vi "FTW-CodeGen-Prototype.vi"(0 "REPLACE_Actor Instance Configuration":string="{\n  \"Identity\": \"ActorName\",\n  \"InboxAddress\": \"tcp://127.0.0.1:*\",\n  \"SupervisorAddress\": \"\",\n  \"DebugEnableInboxLogging\": false,\n  \"DebugEnableJobLogging\": false,\n  \"DebugShowPanel\": false\n}", 2 "ADAPT_Actor Instance Interface":refnum<vi>, 5 "REPLACE_Launch Actor from Filepath":path=path "", 11 "REPLACE_error in":errorcluster) -> (4 "REPLACE_FTW Actor Connector":T1, 6 "REPLACE_Instance Inbox Address":string, 8 "REPLACE_Instance VI Clone Name":string, 15 "REPLACE_error out":errorcluster)   [LabVIEW 2015, in "FTW-Actor-Spawn.xnode"]
uses:
  FTW-Actor-Spawn.xnode
  src/core/type/FTW-Type-Actor-Connector.ctl
  src/error/FTW-ERR-ThrowError.vi
  src/reflection/FTW-Reflection-Type.vi
  src/error/FTW-ERR-NoErrorConstant.vi
  src/error/FTW-ERR-StatusException.vi
  src/error/FTW-ERR-CallChain.vi
  src/string/FTW-STR-ReplaceWhitespace.vi
  src/reflection/FTW-Reflection-Array.vi
  src/string/FTW-STR-Array-Delimit.vi
  src/error/FTW-ERR-Clear.vi
  src/regex/FTW-Regex-ReplaceAll.vi
  lib/FTW-KernelFilepath.vi
  src/json/core/FTW-JSON-Core-EncodingFlags.vi
  json/fetch/FTW-JSON-Core-GetFlattenedValue.vi
  FTW-JSON-Fetch.xnode
panel:
  # "Inputs"
  # "Outputs"
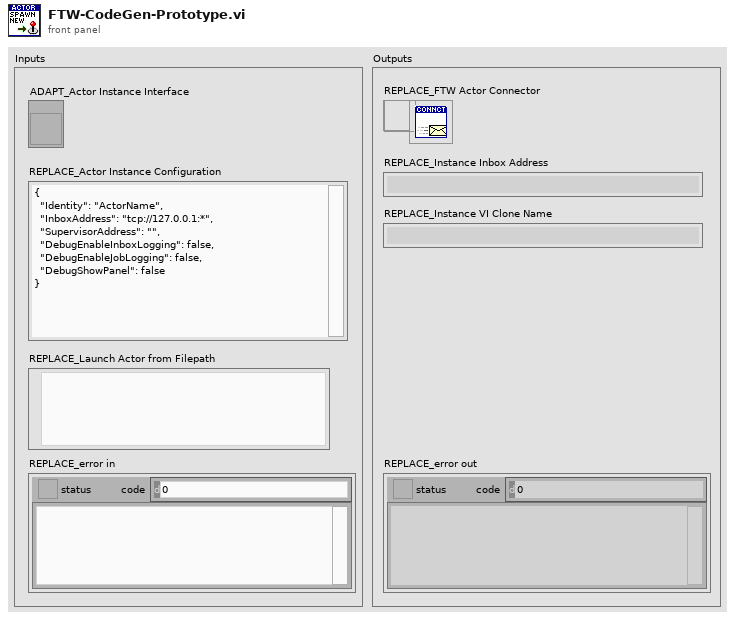
[diagram p1: front panel]
types:
  T1 = typedef "FTW-Type-Actor-Connector.ctl" = refnum<data-value>
  T2 = cluster{"FTW-PrimaryInboxAddress":string, "FTW-InstanceCloneName":string}
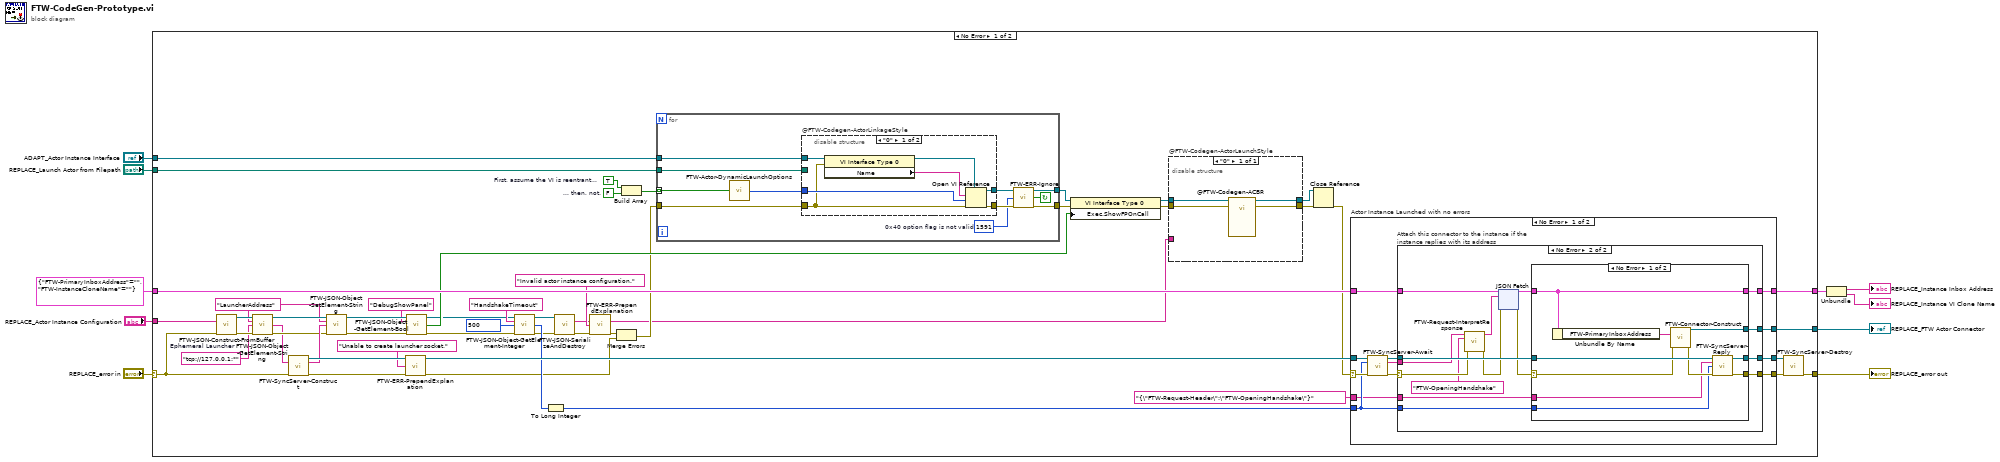
[diagram p0: block diagram]
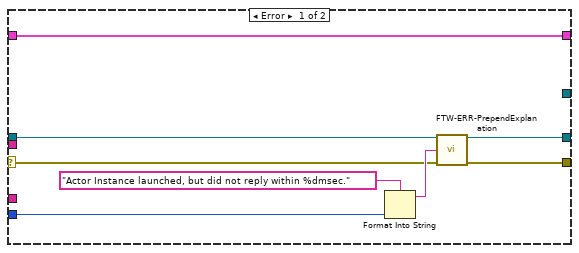
[diagram p2: hidden frame]
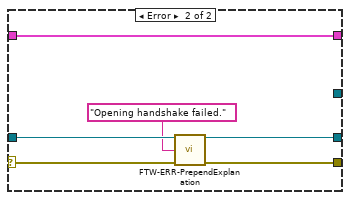
[diagram p3: hidden frame]
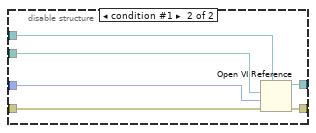
[diagram p5: hidden frame]
diagram:
  n1 = case shown="No Error" "REPLACE_error in" {
    selector: "REPLACE_error in" -> [w37 w202]
    tunnel: [w57 w202] -> w8
    tunnel: [w60 _] -> w9
    tunnel: "REPLACE_Actor Instance Configuration" -> [w40 _]
    tunnel: T2 {"FTW-PrimaryInboxAddress"="", "FTW-InstanceCloneName"=""} -> [w55 w201]
    tunnel: [w54 w201] -> w6
    tunnel: "ADAPT_Actor Instance Interface" -> [w44 _]
    tunnel: "REPLACE_Launch Actor from Filepath" -> [w41 _]
    frame No Error {
      w49 = FALSE  # ... then, not.
      w48 = TRUE  # First, assume the VI is reentrant...
      w13 = "tcp://127.0.0.1:*"  # Ephemeral Launcher
      w11 = "LauncherAddress" ("Key")
      n2 = call "FTW-JSON-Construct-FromBuffer.vi"("JSON String (UTF-8)"=w40, "error in"=w37) -> ("JSON Object"=w17:refnum<data-value>, "error out"=w15:errorcluster)  [unwired: 12 in]
      n3 = call "FTW-JSON-Object-GetElement-String.vi"("JSON Object"=w17, "Key"=w11, "Default Value"=w13, "error in"=w15) -> ("JSON Object out"=w16:refnum<data-value>, "Value"=w12:string, "error out"=w14:errorcluster)  [unwired: 8 in, 1 out]
      n4 = call "FTW-SyncServer-Construct.vi"("Instance Inbox Address"=w12, "error in"=w37) -> ("FTW Synchronous Server"=w56:refnum<data-value>, "Resolved Inbox Address"=w39:string, "error out"=w24:errorcluster)  [unwired: 11 in]
      n5 = call "FTW-JSON-Object-SetElement-String.vi"("JSON Object"=w16, "Key"=w11, "Value"=w39, "error in"=w14) -> ("JSON Object out"=w38:refnum<data-value>, "error out"=w36:errorcluster)  [unwired: 10 in]
      n6 = call "FTW-ERR-PrependExplanation.vi"("Exception Information"="Unable to create launcher socket.", "error in"=w24) -> ("error out"=w23:errorcluster)  [unwired: 13 in]
      n7 = call "FTW-JSON-Object-GetElement-Bool.vi"("JSON Object"=w38, "Key"="DebugShowPanel", "error in"=w36) -> ("JSON Object out"=w32:refnum<data-value>, "Value"=w34:bool, "error out"=w31:errorcluster)  [unwired: 9 in, 1 out]
      n8 = call "FTW-JSON-Object-GetElement-Integer.vi"("JSON Object"=w32, "Key"="HandshakeTimeout", "Default Value"=i64 500, "error in"=w31) -> ("JSON Object out"=w27:refnum<data-value>, "Value"=w30:i64, "error out"=w26:errorcluster)  [unwired: 8 in, 1 out]
      n9 = To Long Integer(number=w30) -> (32bit integer=w29:i32)
      n10 = call "FTW-JSON-SerializeAndDestroy.vi"("JSON Object"=w27, "error in"=w26) -> ("JSON String (UTF-8)"=w18:string, "error out"=w21:errorcluster)  [unwired: 12 in]
      n11 = call "FTW-ERR-PrependExplanation.vi"("Exception Information"="Invalid actor instance configuration.", "error in"=w21) -> ("error out"=w20:errorcluster)  [unwired: 13 in]
      n12 = Merge Errors(w20, w23) -> (w25:errorcluster)
      n13 = Build Array(w48, w49) -> (w50:bool[])
      n14 = for {
        tunnel: w44 -> [w187]
        tunnel: [w185] -> w46
        tunnel: [w181] -> w47
        tunnel: w50 -> [w184] mode=indexing
        tunnel: w25 -> [w183]
        tunnel: w41 -> [w182]
        stop <- w179 continue-if-true
        w178 = 1591  # 0x40 option flag is not valid
        n15 = call "FTW-Actor-DynamicLaunchOptions.vi"("Reentrant?"=w184) -> ("Open VI Ref Options"=w186:i32)
        n16 = disable-structure "@FTW-Codegen-ActorLinkageStyle" shown="\"0\"" {
          disable-tunnel: w187 -> [w194 w200]
          disable-tunnel: w186 -> [w193 w199]
          disable-tunnel: [w192 w198] -> w185
          disable-tunnel: w183 -> [w191 w197]
          disable-tunnel: [w190 w196] -> w180
          disable-tunnel: w182 -> [_ w195]
          frame condition #0 (active) {
            n17 = property class="VI Interface Type 0"(reference=w194, error in=w191) -> (reference out=w189:refnum<vi>, "Name"=w188:string)  [unwired: 1 out]
            n18 = Open VI Reference(type specifier VI Refnum (for type only)=w189, vi path=w188, options=w193, error in (no error)=w191) -> (vi reference=w192:refnum<vi>, error out=w190:errorcluster)  [unwired: 2 in]
          }
          frame condition #1 {
            n19 = Open VI Reference(type specifier VI Refnum (for type only)=w200, vi path=w195, options=w199, error in (no error)=w197) -> (vi reference=w198:refnum<vi>, error out=w196:errorcluster)  [unwired: 2 in]
          }
        }
        n20 = call "FTW-ERR-Ignore.vi"("Error Code"=w178, "error in"=w180) -> ("Error Cleared?"=w179:bool, "error out"=w181:errorcluster)  [unwired: 12 in]
      }
      n21 = property class="VI Interface Type 0"(reference=w46, error in=w47, "Exec.ShowFPOnCall"=w34) -> (reference out=w51:refnum<vi>, error out=w52:errorcluster)
      n22 = disable-structure "@FTW-Codegen-ActorLaunchStyle" shown="\"0\"" {
        disable-tunnel: [w64] -> w53
        disable-tunnel: w52 -> [w63]
        disable-tunnel: w51 -> [w62]
        disable-tunnel: [w61] -> w42
        disable-tunnel: w18 -> [_]
        frame condition #0 (active) {
          n23 = call-by-ref "@FTW-Codegen-ACBR"(reference=w62, error in=w63) -> (reference out=w61:refnum<vi>, error out=w64:errorcluster)  [unwired: 1 in]
        }
      }
      n24 = Close Reference(reference=w42, error in (no error)=w53) -> (error out=w45:errorcluster)
      n25 = case "Actor Instance Launched with no errors" shown="No Error" w45 {
        selector: w45 -> [w71 w177]
        tunnel: [w76 w177] -> w58
        tunnel: [w75 _] -> w60
        tunnel: w56 -> [w73 w176]
        tunnel: [w74 w176] -> w59
        tunnel: [w66 w175] -> w54
        tunnel: w29 -> [w69 _]
        tunnel: w55 -> [w67 w175]
        tunnel: "{\"FTW-Request-Header\":\"FTW-OpeningHandshake\"}" -> [w65 _]
        frame No Error {
          n26 = call "FTW-SyncServer-Await.vi"("FTW Synchronous Server"=w73, "Receive Timeout"=w69, "error in"=w71) -> ("FTW Synchronous Server out"=w72:refnum<data-value>, "Incoming Request"=w68:string, "error out"=w70:errorcluster)  [unwired: 10 in]
          n27 = case "Attach this connector to the instance if the instance replies with its address" shown="No Error" w70 {
            selector: w70 -> [w78 w92]
            tunnel: [w77 w97] -> w76
            tunnel: [_ w98] -> w75
            tunnel: w72 -> [w83 w94]
            tunnel: [w83 w95] -> w74
            tunnel: w69 -> [w81 w96]
            tunnel: w68 -> [_ w91]
            tunnel: w67 -> [w80 w89]
            tunnel: [w80 w93] -> w66
            tunnel: w65 -> [_ w84]
            frame Error {
              n28 = Format Into String(format string="Actor Instance launched, but did not reply within %dmsec." ("Error Message"), w81) -> (resulting string=w79:string)  [unwired: 2 in, 1 out]
              n29 = call "FTW-ERR-PrependExplanation.vi"("Exception Information"=w79, "error in"=w78) -> ("error out"=w77:errorcluster)  [unwired: 13 in]
            }
            frame No Error {
              n30 = call "FTW-Request-InterpretResponse.vi"("Raw Request"=w91, "Request Header"="FTW-OpeningHandshake", "error in"=w92) -> ("JSON Response"=w85:string, "error out"=w87:errorcluster)  [unwired: 11 in]
              n31 = xnode "JSON Fetch"("Type and Defaults"=w89, "JSON String"=w85, "error in"=w87) -> ("Values"=w88:T2, "error out"=w86:errorcluster)  [unwired: 1 in]
              n32 = case shown="No Error" w86 {
                selector: w86 -> [w163 w171]
                tunnel: [w169 _] -> w98
                tunnel: [w161 w174] -> w97
                tunnel: w88 -> [w165 w172]
                tunnel: w94 -> [w167 w173]
                tunnel: w96 -> [w164 _]
                tunnel: [w162 w173] -> w95
                tunnel: [w165 w172] -> w93
                tunnel: w84 -> [w160 _]
                frame No Error {
                  n33 = Unbundle By Name(w165) -> ("FTW-PrimaryInboxAddress"=w168:string)
                  n34 = call "FTW-Connector-Construct.vi"("Remote Inbox Address"=w168, "error in"=w163) -> ("FTW Actor Connector"=w169:T1, "error out"=w166:errorcluster)  [unwired: 12 in]
                  n35 = call "FTW-SyncServer-Reply.vi"("FTW Synchronous Server"=w167, "Response"=w160, "Send Timeout"=w164, "error in"=w166) -> ("FTW Synchronous Server out"=w162:refnum<data-value>, "error out"=w161:errorcluster)  [unwired: 10 in]
                }
                frame Error {
                  n36 = call "FTW-ERR-PrependExplanation.vi"("Exception Information"="Opening handshake failed.", "error in"=w171) -> ("error out"=w174:errorcluster)  [unwired: 13 in]
                }
              }
            }
          }
        }
        frame Error {
        }
      }
      n37 = call "FTW-SyncServer-Destroy.vi"("FTW Synchronous Server"=w59, "error in"=w58) -> ("error out"=w57:errorcluster)  [unwired: 13 in]
    }
    frame Error {
    }
  }
  "REPLACE_error out" <- w8
  "REPLACE_FTW Actor Connector" <- w9
  n38 = Unbundle(w6) -> ("FTW-PrimaryInboxAddress"=→"REPLACE_Instance Inbox Address":string, "FTW-InstanceCloneName"=→"REPLACE_Instance VI Clone Name":string)
